vi "ROI entry-Previous ROI load.vi"() -> (1 "Proceed":bool)   [LabVIEW 2020]
uses:
  Typedefs/ROI management FG states.ctl
  <userlib>/My Palettes.lib/Files & paths/Spreadsheet/Read From Spreadsheet File (DBL)-Mod.vi
  Globals/gl_ROI Entry UI globals.vi
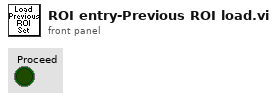
[diagram p1: front panel]
types:
  T1 = typedef "ROI fitting info cluster.ctl" = cluster{"ROI fit info":cluster{"Fit ROI to new frame size":bool, "Frame size":cluster{"Old":T2, "New":T2}}, "Adjust Motor Z":bool}
  T2 = typedef "Frame Size.ctl" = u16
  T3 = typedef "ROI ID Enum.ctl" = enum16{"Point", "MiniScan", "Comp. MiniScan", "Rectangle", "Comp. volume", "Arb. plane point", "None"}
  T4 = typedef "ROI management FG states.ctl" = enum16{"Read", "Write", "Write-from dataset", "Clear Last", "Clear All", "Delete ROI", "Update ROIs time", "Reload last ROI set", "Modify ROI Parameters", "Offset all ROI", "Offset visible ROI", "Modify Dwell Time", "Modify Laser Power"}
  T5 = enum8{"Enabled", "Disabled", "Disabled and Grayed Out"}
  T6 = typedef "ROI parameters data type.ctl" = cluster{"ROI index":dbl, "ROI ID":dbl, "ROI Time (ns)":dbl, "Pixels in ROI":dbl, "X start":dbl, "Y start":dbl, "Z start":dbl, "X stop":dbl, "Y stop":dbl, "Z stop":dbl, "Angle (deg)":dbl, "Composite ID":dbl, "Number of lines":dbl, "Frame Size":dbl, "Zoom":dbl, "Laser Power (%)":dbl, "ROI group ID":dbl, "Resolution":dbl, "Dwell Time per pixel":dbl, "Pixels per miniscan":dbl, "Original FOV (um)":dbl, "Apparent Frame Size":dbl, "Z Plane Idx":i32[], "Z Plane codes":i32[]}
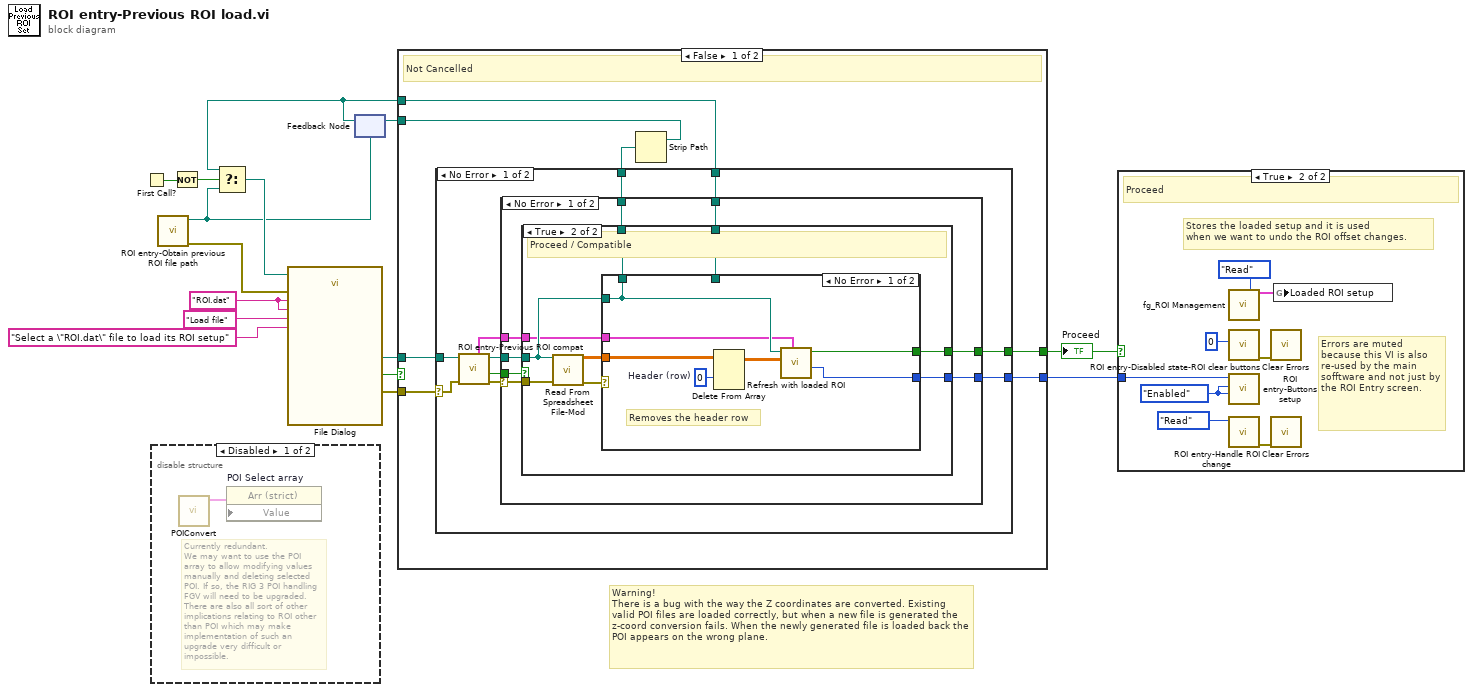
[diagram p0: block diagram]
diagram:
  w13 = "ROI.dat" ("pattern (all files)")
  # "Warning!\nThere is a bug with the way the Z coordinates are converted. Existing valid POI files are loaded correctly, but when a new file is generated the z-coord conversion fails. When the newly generated file is loaded back the POI appears on the wrong plane."
  n1 = First Call?() -> (First Call?: T/F=w8:bool)
  n2 = disable-structure shown="Disabled" {
    frame Disabled {
      # "Currently redundant.\nWe may want to use the POI array to allow modifying values manually and deleting selected POI. If so, the RIG 3 POI handling FGV will need to be upgraded. There are also all sort of other implications relating to ROI other than POI which may make implementation of such an upgrade very difficult or impossible."
      n3 = call "POIConvert.vi"() -> ("POISelectArrayOut"=w16:cluster{"System Array":dbl[], "Boolean":bool}[])  [unwired: 11 in]
      n4 = property on="POI Select array" class="Arr (strict)"("Value"=w16) -> ()  [unwired: 2 in, 2 out]
    }
    frame Enabled {
    }
  }
  n5 = call "ROI entry-Obtain previous ROI file path.vi"() -> ("error out"=w2:errorcluster, "Experiment folder path containing last ROI file"=w1:path)  [unwired: 10 in]
  n6 = Not(x=w8) -> (.not. x?=w9:bool)
  n7 = feedback #1(w1) -> (w11:path)
  n8 = Select(t=w11, s=w9, f=w1) -> (s? t:f=w10:path)
  n9 = call "File Dialog"("start path"=w10, "prompt"="Select a \"ROI.dat\" file to load its ROI setup", "button label"="Load file", "error in"=w2, "pattern (all files)"=w13, "pattern label"=w13) -> ("selected path"=w5:path, "cancelled"=w7:bool, "error out"=w6:errorcluster)  [unwired: 6 in, 1 out]
  n10 = case shown="False" w7 {
    tunnel: w5 -> [w23 _]
    tunnel: w6 -> [w22 _]
    tunnel: w11 -> [w19 w62]
    tunnel: [w20 w62] -> w12
    tunnel: [w18 _] -> w3
    tunnel: [w17 _] -> w4
    frame False {
      # "Not Cancelled"
      n11 = case shown="No Error" w22 {
        selector: w22 -> [w29 _]
        tunnel: w23 -> [w26 _]
        tunnel: [w33 w61] -> w21
        tunnel: w19 -> [w32 w61]
        tunnel: [w31 _] -> w18
        tunnel: [w30 _] -> w17
        frame No Error {
          n12 = call "ROI entry-Previous ROI compat.vi"("error in (no error)"=w29, "Old ROI file path"=w26) -> ("error out"=w28:errorcluster, "Proceed"=w27:bool, "Old ROI file path (dup)"=w25:path, "ROI fit info cluster"=w24:T1)  [unwired: 6 in]
          n13 = case shown="No Error" w28 {
            selector: w28 -> [w36 _]
            tunnel: [w41 w60] -> w33
            tunnel: w32 -> [w40 w60]
            tunnel: w25 -> [w39 _]
            tunnel: [w38 _] -> w31
            tunnel: [w37 _] -> w30
            tunnel: w27 -> [w35 _]
            tunnel: w24 -> [w34 _]
            frame No Error {
              n14 = case shown="True" w35 {
                tunnel: [w42 w49] -> w41
                tunnel: w40 -> [w42 w48]
                tunnel: w39 -> [_ w47]
                tunnel: [_ w46] -> w38
                tunnel: [_ w45] -> w37
                tunnel: w36 -> [_ w44]
                tunnel: w34 -> [_ w43]
                frame False {
                  # "Cancelled / Incompatible"
                }
                frame True {
                  # "Proceed / Compatible"
                  n15 = call-poly <userlib>:"Read From Spreadsheet File-Mod.vi"("file path (dialog if empty)"=w47, "error in"=w44) -> ("all rows"=w51:dbl[][], "error out"=w50:errorcluster)  [unwired: 8 in, 4 out]
                  n16 = case shown="No Error" w50 {
                    tunnel: w51 -> [w58 _]
                    tunnel: [w53 w59] -> w49
                    tunnel: w48 -> [_ w59]
                    tunnel: w47 -> [w53 _]
                    tunnel: [w57 _] -> w46
                    tunnel: [w56 _] -> w45
                    tunnel: w43 -> [w52 _]
                    frame No Error {
                      w54 = 0  # Header (row)
                      # "Removes the header row"
                      n17 = Delete From Array(array=w58, index (row)=w54) -> (array with subset deleted=w55:dbl[][])  [unwired: 2 in, 1 out]
                      n18 = call "Refresh with loaded ROI.vi"("ROI fit info cluster"=w52, "Old ROI file's data"=w55, "Old ROI file path"=w53) -> ("Last ROI Enum"=w56:T3, "Proceed?"=w57:bool)  [unwired: 7 in]
                    }
                    frame Error {
                    }
                  }
                }
              }
            }
            frame Error {
            }
          }
        }
        frame Error {
        }
      }
      n19 = Strip Path(path=w21) -> (stripped path=w20:path)  [unwired: 1 out]
    }
    frame True {
      # "Cancelled"
    }
  }
  "Proceed" <- w3
  n20 = feedback-in #1(w12) -> ()
  n21 = case shown="True" w3 {
    tunnel: w4 -> [_ w63]
    frame False {
      # "Do not proceed"
    }
    frame True {
      w64 = T5."Enabled" ("Done button disabled?")
      # "Stores the loaded setup and it is used\nwhen we want to undo the ROI offset changes."
      # "Errors are muted because this VI is also re-used by the main sofftware and not just by the ROI Entry screen."
      # "Proceed"
      n22 = call "fg_ROI Management.vi"("Function"=ROI_management_FG_states."Read") -> ("ROI Setup"=w65:T6[])  [unwired: 8 in, 6 out]
      n23 = call "ROI entry-Disabled state-ROI clear buttons.vi"("State"=0) -> ("error out"=w69:errorcluster)  [unwired: 10 in]
      n24 = call "ROI entry-Buttons setup.vi"("Acquisition button disabled?"=w64, "Done button disabled?"=w64, "ROI Enum"=w63) -> ()  [unwired: 9 in]
      n25 = call "ROI entry-Handle ROI change.vi"("ROI management"=ROI_management_FG_states."Read") -> ("error out"=w68:errorcluster)  [unwired: 8 in, 2 out]
      n26 = call <vilib>:"Clear Errors.vi"("error in (no error)"=w69) -> ()  [unwired: 5 in, 2 out]
      n27 = call <vilib>:"Clear Errors.vi"("error in (no error)"=w68) -> ()  [unwired: 5 in, 2 out]
      n28 = global write "gl_ROI Entry UI globals.vi" "Loaded ROI setup"(w65) -> ()
    }
  }
